vi "DriveRamp.vi"(1 "dt (s)":dbl, 2 "Setpoint X (mv)":dbl, 3 "Ramp Time (s)":dbl) -> (0 "Ramped Output X (mv)":dbl)   [LabVIEW 2014]
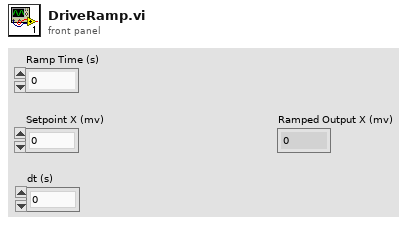
[diagram p1: front panel]
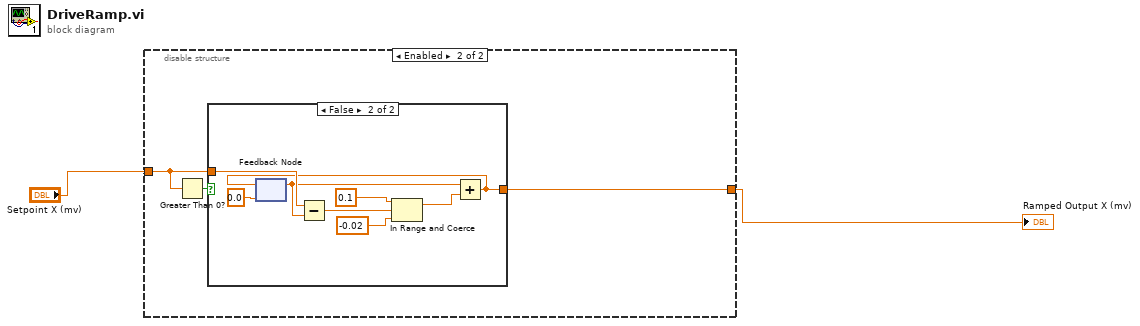
[diagram p0: block diagram]
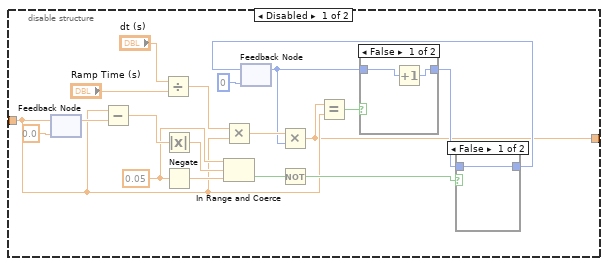
[diagram p2: hidden frame]
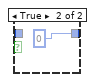
[diagram p3: hidden frame]
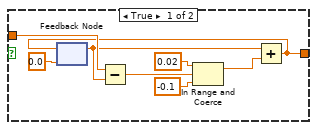
[diagram p5: hidden frame]
diagram:
  n1 = disable-structure shown="Enabled" {
    disable-tunnel: "Setpoint X (mv)" -> [w4 w27]
    disable-tunnel: [w3 w29] -> w1
    frame Disabled {
      w11 = 0.05
      n2 = feedback #1(0.0) -> (w14:dbl)
      n3 = feedback-in #1(w4) -> ()
      n4 = Subtract(x=w4, y=w14) -> (x-y=w13:dbl)
      n5 = Divide(x="dt (s)", y="Ramp Time (s)") -> (x/y=w9:dbl)
      n6 = Absolute Value(x=w13) -> (abs(x)=w12:dbl)
      n7 = Negate(x=w11) -> (-x=w10:dbl)
      n8 = Multiply(x=w9, y=w4) -> (x*y=w21:dbl)
      n9 = In Range and Coerce(upper limit=w11, x=w12, lower limit=w10) -> (In Range?=w6:bool)  [unwired: 1 out]
      n10 = feedback #2(0) -> (w19:i32)
      n11 = Multiply(x=w21, y=w19) -> (x*y=w3:dbl)
      n12 = Not(x=w6) -> (.not. x?=w5:bool)
      n13 = Equal?(x=w3, y=w4) -> (x = y?=w18:bool)
      n14 = case shown="False" w18 {
        tunnel: w19 -> [w25 w26]
        tunnel: [w24 w26] -> w16
        frame False {
          n15 = Increment(x=w25) -> (x+1=w24:i32)
        }
        frame True {
        }
      }
      n16 = case shown="False" w5 {
        tunnel: w16 -> [w22 _]
        tunnel: [w22 0] -> w15
        frame False {
        }
        frame True {
        }
      }
      n17 = feedback-in #2(w15) -> ()
    }
    frame Enabled {
      n18 = Greater Than 0?(x=w27) -> (x > 0?=w28:bool)
      n19 = case shown="False" w28 {
        tunnel: w27 -> [w32 w41]
        tunnel: [w30 w39] -> w29
        frame True {
          n20 = feedback #3(0.0) -> (w31:dbl)
          n21 = Subtract(x=w32, y=w31) -> (x-y=w36:dbl)
          n22 = In Range and Coerce(upper limit=0.02, x=w36, lower limit=-0.1) -> (coerced(x)=w33:dbl)  [unwired: 1 out]
          n23 = Add(x=w31, y=w33) -> (x+y=w30:dbl)
          n24 = feedback-in #3(w30) -> ()
        }
        frame False {
          n25 = feedback #4(0.0) -> (w40:dbl)
          n26 = Subtract(x=w41, y=w40) -> (x-y=w44:dbl)
          n27 = In Range and Coerce(upper limit=0.1, x=w44, lower limit=-0.02) -> (coerced(x)=w42:dbl)  [unwired: 1 out]
          n28 = Add(x=w40, y=w42) -> (x+y=w39:dbl)
          n29 = feedback-in #4(w39) -> ()
        }
      }
    }
  }
  "Ramped Output X (mv)" <- w1
